vi "dfd_Build Tag.vi"(11 "element name":string) -> (1 "empty tag":string, 2 "end tag":string, 3 "start tag":string)   [LabVIEW 2017, in "NI_DigFilter_Process.lvlib"]
uses:
  <vilib>/addons/Digital Filter Design/NI_DigFilter_Process.lvlib
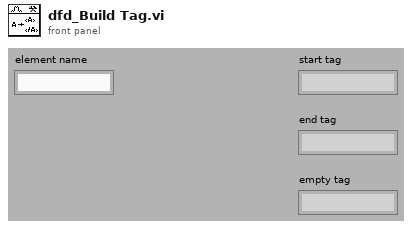
[diagram p1: front panel]
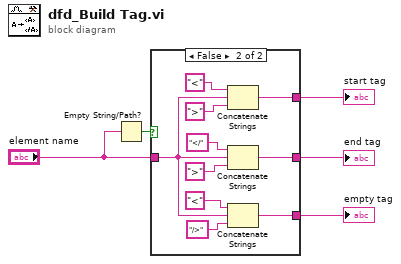
[diagram p0: block diagram]
diagram:
  n1 = Empty String/Path?(string/path="element name") -> (empty?=w3:bool)
  n2 = case shown="False" w3 {
    tunnel: [_ w11] -> w5
    tunnel: [_ w10] -> w4
    tunnel: "element name" -> [_ w7]
    tunnel: [_ w6] -> w1
    frame True {
    }
    frame False {
      n3 = Concatenate Strings("<", w7, ">") -> (w10:string)
      n4 = Concatenate Strings("</", w7, ">") -> (w11:string)
      n5 = Concatenate Strings("<", w7, "/>") -> (w6:string)
    }
  }
  "start tag" <- w4
  "end tag" <- w5
  "empty tag" <- w1
